vi "compare config files.vi"() -> ()   [LabVIEW 2011]
uses:
  <vilib>/Utility/file.llb/Read From Spreadsheet File (string).vi
panel:
  out "Array":string[][](array[string])
  in  "file path (dialog if empty) 2":path
  in  "file path (dialog if empty)":path
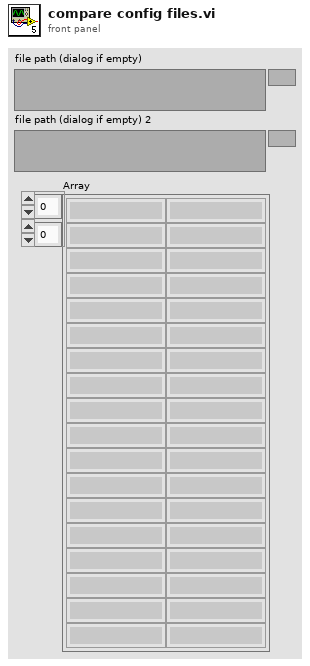
[diagram p1: front panel]
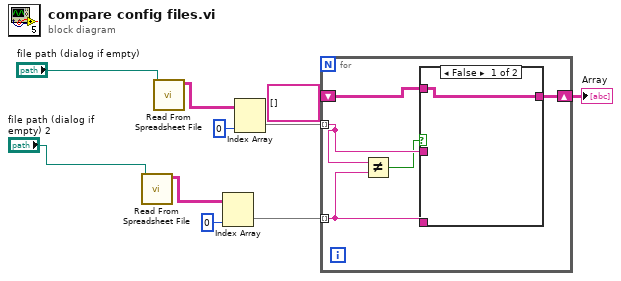
[diagram p0: block diagram]
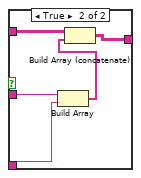
[diagram p2: hidden frame]
diagram:
  n1 = call-poly <vilib>:"Read From Spreadsheet File.vi"("file path (dialog if empty)"="file path (dialog if empty) 2") -> ("all rows"=w6:string[][])  [unwired: 6 in, 4 out]
  n2 = call-poly <vilib>:"Read From Spreadsheet File.vi"("file path (dialog if empty)"="file path (dialog if empty)") -> ("all rows"=w9:string[][])  [unwired: 6 in, 4 out]
  n3 = Index Array(array=w6, index (col)=0 ("disabled index (col)")) -> (element=w4:string[])  [unwired: 1 in]
  n4 = Index Array(array=w9, index (col)=0 ("disabled index (col)")) -> (element=w3:string[])  [unwired: 1 in]
  n5 = for {
    tunnel: w4 -> [w14] mode=indexing
    tunnel: w3 -> [w15] mode=indexing
    shift-right: [w13] -> w1
    shift-left: string[][] [] -> [w12]
    n6 = Not Equal?(x=w15, y=w14) -> (x != y?=w11:bool)
    n7 = case shown="False" w11 {
      tunnel: w15 -> [_ w21]
      tunnel: w14 -> [_ w20]
      tunnel: [w16 w18] -> w13
      tunnel: w12 -> [w16 w17]
      frame False {
      }
      frame True {
        n8 = Build Array(w21, w20) -> (w19:string[])
        n9 = Build Array (concatenate)(w17, w19) -> (w18:string[][])
      }
    }
  }
  "Array" <- w1
